vi "Configure Edge Trigger Source.vi"(7 "Trigger Slope (Positive)":i32(slide), 8 "error in (no error)":errorcluster {"code" format="%.0x"}, 9 "Trigger Level (0.0 V)":dbl format="%.2p", 10 "Trigger Source (Channel 1)":string(combo)="CH1", 11 "VISA Resource Name":refnum<visa-resource-name>) -> (0 "error out":errorcluster {"code" format="%.0x"}, 3 "VISA Resource Name Out":refnum<visa-resource-name>)   [LabVIEW 2010, in "Tektronix TDS 3000 Series.lvlib"]
doc: "This VI configures the edge trigger. An edge trigger occurs when the trigger signal passes through the voltage threshold that you specify with the Trigger Level control and has the slope that you specify with the Trigger Slope control. \n\nNotes:\n\n(1) This VI affects instrument behavior only if the Trigger Type is Edge Trigger. Call the Configure Trigger VI to set the Trigger Type before you call this VI."
uses:
  <instrlib>/Tektronix TDS 3000 Series/Tektronix TDS 3000 Series.lvlib
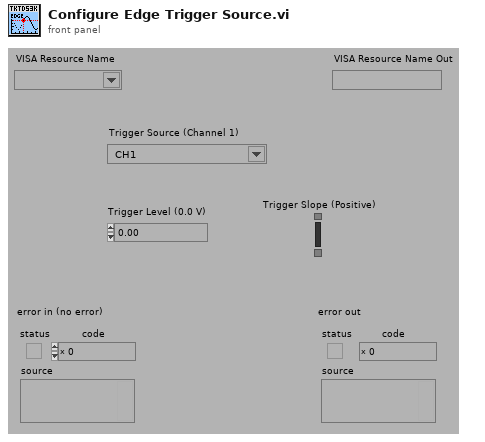
[diagram p1: front panel]
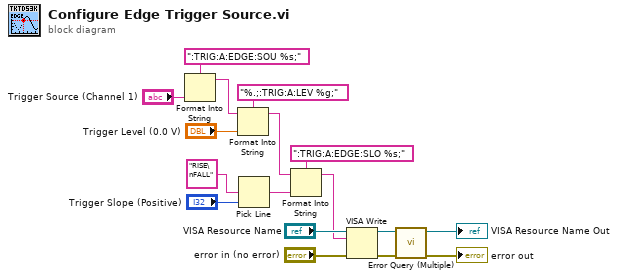
[diagram p0: block diagram]
diagram:
  n1 = Format Into String(format string=":TRIG:A:EDGE:SOU %s;", "Trigger Source (Channel 1)") -> (resulting string=w6:string)  [unwired: 2 in, 1 out]
  n2 = Format Into String(format string="%.;:TRIG:A:LEV %g;", initial string=w6, "Trigger Level (0.0 V)") -> (resulting string=w7:string)  [unwired: 1 in, 1 out]
  n3 = Pick Line(multi-line string="RISE\nFALL", line index="Trigger Slope (Positive)") -> (output string=w9:string)  [unwired: 1 in]
  n4 = Format Into String(format string=":TRIG:A:EDGE:SLO %s;", initial string=w7, w9) -> (resulting string=w5:string)  [unwired: 1 in, 1 out]
  n5 = VISA Write(VISA resource name="VISA Resource Name", write buffer=w5, error in (no error)="error in (no error)") -> (VISA resource name out=w4:refnum<visa-resource-name>, error out=w3:errorcluster)  [unwired: 1 out]
  n6 = call <instrlib>:"Error Query (Multiple).vi"("error in (no error)"=w3, "VISA Resource Name"=w4) -> ("error out"=→"error out":errorcluster, "VISA Resource Name Out"=→"VISA Resource Name Out":refnum<visa-resource-name>)  [unwired: 6 in, 2 out]
